vi "recipeScript repeatFile.vi"(8 "error in (no error)":errorcluster, 11 "path":path) -> (0 "error out":errorcluster, 3 "dup path":path)   [LabVIEW 2018]
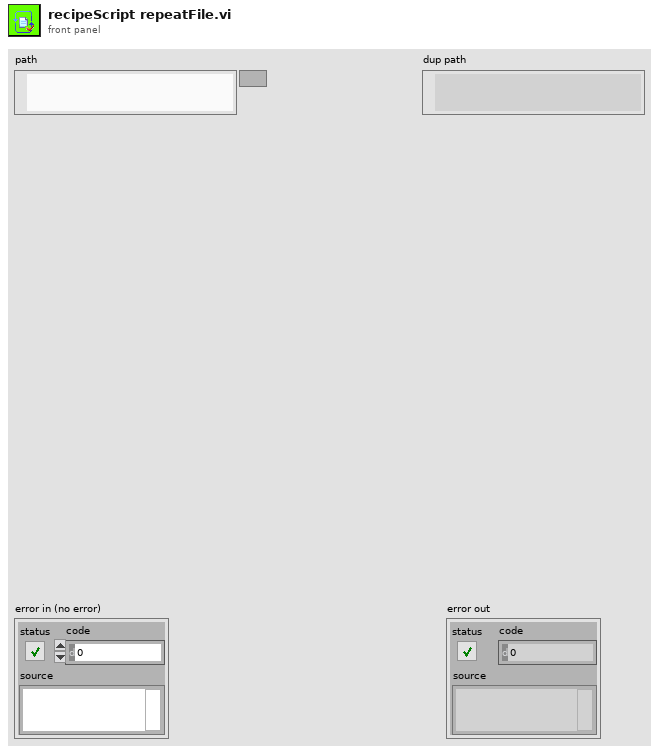
[diagram p1: front panel]
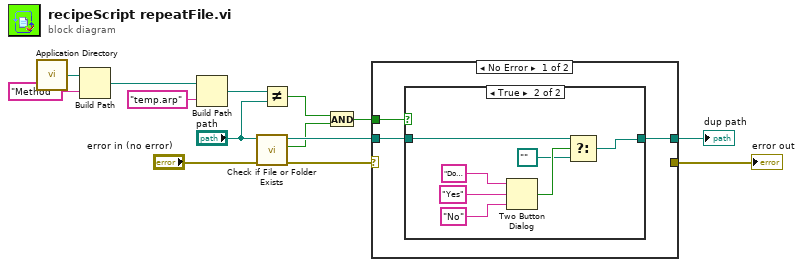
[diagram p0: block diagram]
diagram:
  n1 = call <vilib>:"Application Directory.vi"() -> ("Application Directory"=w9:path)
  n2 = Build Path(base path=w9, name or relative path="Method") -> (appended path=w7:path)
  n3 = Build Path(base path=w7, name or relative path="temp.arp") -> (appended path=w5:path)
  n4 = call <vilib>:"Check if File or Folder Exists.vi"("error in (no error)"="error in (no error)", "path"="path") -> ("error out"=w13:errorcluster, "file or folder exists?"=w2:bool, "dup path"=w12:path)  [unwired: 7 in]
  n5 = Not Equal?(x=w5, y="path") -> (x != y?=w3:bool)
  n6 = And(x=w3, y=w2) -> (x .and. y?=w1:bool)
  n7 = case shown="No Error" w13 {
    selector: w13 -> [_ w26]
    tunnel: w1 -> [w17 _]
    tunnel: w12 -> [w16 _]
    tunnel: [w15 _] -> w11
    tunnel: [_ w26] -> w10
    frame No Error {
      n8 = case shown="True" w17 {
        tunnel: w16 -> [w18 w21]
        tunnel: [w18 w19] -> w15
        frame False {
        }
        frame True {
          n9 = Two Button Dialog(message="Do you want to overwrite this file?", 1:"No" ("F button name (\"Cancel\")"), 2:"Yes" ("T button name (\"OK\")")) -> (T button?=w22:bool)
          n10 = Select(t=w21, s=w22, f=path "") -> (s? t:f=w19:path)
        }
      }
    }
    frame Error {
    }
  }
  "dup path" <- w11
  "error out" <- w10
